vi "Manual Shooter Mode.vi"(8 "Shooter Angle":dbl format="%.2f", 10 "Manual Shoot":T1) -> (0 "Shooter Ready?":bool, 1 "Trigger Output":dbl, 2 "Right Output":dbl, 3 "Left Output":dbl, 4 "Angle Motor Out":dbl)   [LabVIEW 2015]
uses:
  Common Code/Manual Shoot.ctl
  Common Code/Change Detect Double.vi
  Robot Global Data.vi
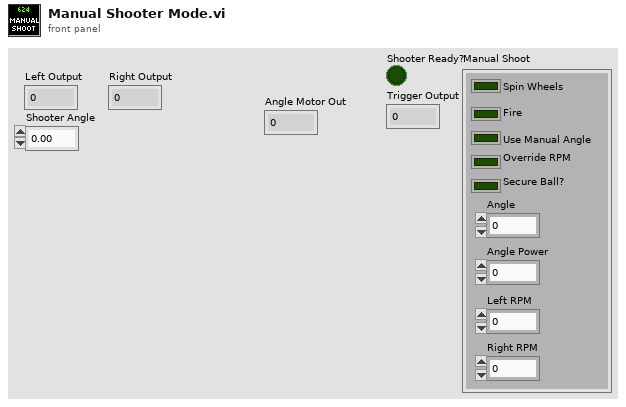
[diagram p1: front panel]
types:
  T1 = typedef "Manual Shoot.ctl" = cluster{"Spin Wheels":bool, "Fire":bool, "Angle":dbl, "Angle Power":dbl, "Use Manual Angle":bool, "Override RPM":bool, "Left RPM":dbl, "Right RPM":dbl, "Secure Ball?":bool}
  T2 = typedef "Dashboard Control Data.ctl" = cluster{"Shooter Presets":T3, "Encoder Control":T5, "Steer PID output":cluster{"output high":dbl, "output low":dbl}, " Steer PID gains":cluster{"proportional gain (Kc)":dbl, "integral time (Ti, min)":dbl, "derivative time (Td, min)":dbl}, "Drivetrain Settings":T6, "Vision Packet":T7, "Dashboard Drivetrain Command":T8, "Info/Command Cluster":T10, "Ball Vision Packet":T11, "Intake Presets":T13, "Intake Encoder Control":T15, "Climb Presets":T16, "Goal Output Range":cluster{"output high":dbl, "output low":dbl}, "Enabled Systems":T17, "Auton Presets":T18, "Pressure M":dbl, "Pressure B":dbl}
  T3 = typedef "Shooter Presets.ctl" = cluster{"Batter Shot":T4, "Deep Middle":T4, "Manual Shot":T4, "Left Ticks Per Rotation":dbl, "Right Ticks Per Rotation":dbl, "Low Bar Shot":T4, "Shooter RPM Tolerance":dbl, "Trigger Power":dbl, "Fire from Load Delay":i32, "Max Angle":dbl, "Min Angle":dbl, "Angle PID gains":cluster{"P":dbl, "I":dbl, "D":dbl}, "Angle Output":cluster{"output high":dbl, "output low":dbl}, "Shooter Angle Tolerance":dbl, "Vision Shoot x^2":dbl, "Vision Shoot x":dbl, "IR Let Go Timer":dbl, "Feed Forward Max Accel":dbl, "Feed Forward Kv":dbl, "Backwards Trigger":dbl, "Shot Finish Delay (ms)":dbl, "Angle Max Current":dbl, "Angle Current Trip Time":dbl, "Intake Angle":dbl, "Vision Shoot c":dbl, "Reset?":bool, "Button Release Delay":dbl, "Angle Pot x":dbl, "Angle Pot c":dbl, "Ignore Angle?":bool, "Max RPM":dbl, "Safty Frist Angle":dbl, "Intake Danger Height":dbl, "Angle Pot B":i32, "Angle Pot M":dbl, "FF Finish RPM":dbl, "RPM PID Right":cluster{"P":dbl, "I":dbl, "D":dbl, "FF":dbl}, "RPM PID Left":cluster{"P":dbl, "I":dbl, "D":dbl, "FF":dbl}, "Backwards RPM":dbl, "Vision RPM":dbl, "Run Wheels Backward Delay":u32, "Cleat Shot":T4}
  T4 = typedef "Shot Presets.ctl" = cluster{"L":dbl, "R":dbl, "A":dbl}
  T5 = typedef "Encoder Control.ctl" = cluster{"Right Tick Constant":dbl, "Left Tick Constant":dbl, "Reset?":bool, "Y Dist":cluster{"PID gains":cluster{"proportional gain (Kc)":dbl, "integral time (Ti, min)":dbl, "derivative time (Td, min)":dbl}}, "Y Stop Thresh":dbl, "Y Stop Speed":dbl}
  T6 = typedef "Drivetrain Settings.ctl" = cluster{"Gyro Tolerance":dbl, "Throttle Ramp (ms)":dbl, "Kv":dbl, "Ka":dbl, "Feed Forward P":dbl, "Feed Forward D":dbl, "Goal Vision PID gains":cluster{"proportional gain (Kc)":dbl, "integral time (Ti, min)":dbl, "derivative time (Td, min)":dbl}, "Goal Detection Window":dbl, "Creep Rate":dbl, "Vision Throttle Threshold":dbl, "Min Turn Output":dbl, "Left Batter Angle":dbl, "Right Batter Angle":dbl}
  T7 = typedef "Goal Vision Packet.ctl" = cluster{"Distance":dbl, "Center X":dbl, "Center Y":dbl, "Found Target?":bool, "Robot Center":dbl, "Angle":dbl}
  T8 = typedef "Dashboard Drivetrain Command.ctl" = cluster{"Drivetrain Vision":T9}
  T9 = typedef "Drivetrain Vision.ctl" = cluster{"Goal Window":dbl, "Ball Window":dbl}
  T10 = typedef "Ball Tracking Command Cluster.ctl" = cluster{"Distance to Ball":dbl, "Desired Angle":dbl, "Command":enum16{"Turn to Ball", "Turn to Angle", "Get Distance"}, "Pixels from Center":dbl}
  T11 = typedef "Ball Vision Packet.ctl" = cluster{"Ball Detected?":bool, "Distance to Ball":dbl, "Desired Angle":dbl, "Pixels from Center":dbl, "Tracking mode":T12}
  T12 = typedef "Tracking Mode.ctl" = enum16{"Turn to Ball", "Turn to Angle"}
  T13 = typedef "Intake Presets.ctl" = cluster{"Intake Speed":dbl, "Outake Speed":dbl, "Low Height":dbl, "Half Height":dbl, "Full Height":dbl, "Angle Speed":dbl, "Angle Tolerance":dbl, "Encoder Scale":dbl, "Load Height":dbl, "Output Range":T14, "Rotation Power Max/Min":dbl, "MaxCurrent":dbl, "Intake Trip Time":dbl, "Idle Height":dbl, "Max Height":dbl, "Reset Encoders?":bool, "PID gains":cluster{"proportional gain (Kc)":dbl, "integral time (Ti, min)":dbl, "derivative time (Td, min)":dbl}, "Intake Stop Delay":u32, "Settle Time":dbl, "Settle Wait Time":dbl}
  T14 = typedef "Drivetrain Output Range.ctl" = cluster{"output high":dbl, "output low":dbl}
  T15 = typedef "IntakeEcoderControl.ctl" = cluster{"Arm Tick Constant":dbl, "Reset?":bool, "Y Dist":cluster{"PID gains":cluster{"proportional gain (Kc)":dbl, "integral time (Ti, min)":dbl, "derivative time (Td, min)":dbl}}, "Y Stop Thresh":dbl, "Y Stop Speed":dbl}
  T16 = typedef "Climb Presets.ctl" = cluster{"Pull Power":dbl, "Extend Power":dbl}
  T17 = typedef "Enabled Systems.ctl" = cluster{"Shoot":bool, "Intake":bool, "DT":bool, "Gyro":bool, "100ms":bool, "US":bool}
  T18 = typedef "Autonomous Presets.ctl" = cluster{"Pitch Limit":dbl, "Roll Limit":dbl, "Start Position":dbl, "Cross Position":dbl}
  T19 = typedef "Intake Status Cluster.ctl" = cluster{"Roller Power":dbl, "Angle Power":dbl, "Intake Mode":T20, "Intake States":T21, "Rollers Active?":bool, "Current Height":dbl, "Target Height":dbl, "Encoder Raw Position":dbl, "Forward Tripped?":bool, "Backward Tripped?":bool, "Override IR?":bool}
  T20 = typedef "Intake Mode.ctl" = enum16{"Safe", "Auto", "Manual"}
  T21 = typedef "Intake States.ctl" = enum16{"Idle", "Set roller speed", "Move to angle", "Go Hard or Go Home", "Ball Settle"}
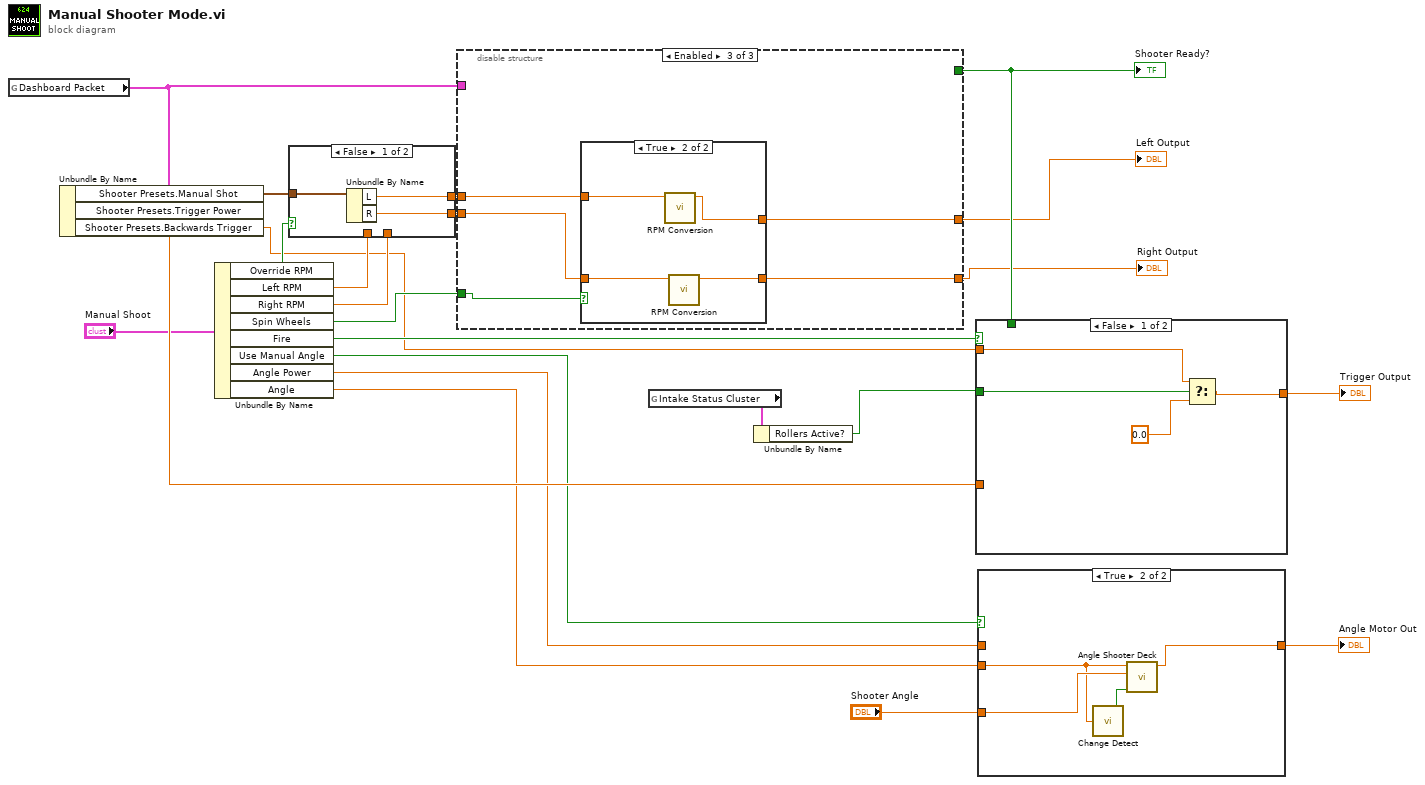
[diagram p0: block diagram]
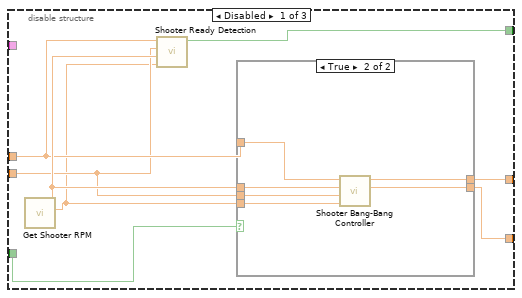
[diagram p2: hidden frame]
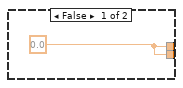
[diagram p3: hidden frame]
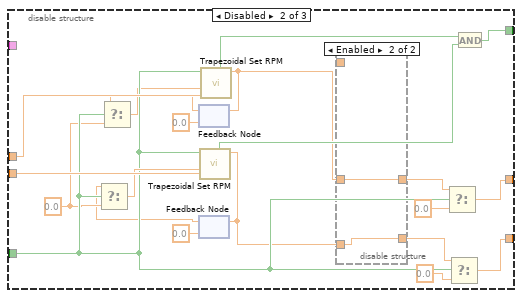
[diagram p4: hidden frame]
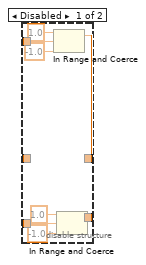
[diagram p5: hidden frame]
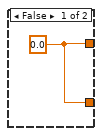
[diagram p6: hidden frame]
diagram:
  n1 = global read "Robot Global Data.vi" "Dashboard Packet"() -> (w2:T2)
  n2 = Unbundle By Name(w2) -> ("Shooter Presets.Manual Shot"=w23:T4, "Shooter Presets.Trigger Power"=w16:dbl, "Shooter Presets.Backwards Trigger"=w7:dbl)
  n3 = Unbundle By Name("Manual Shoot") -> ("Override RPM"=w11:bool, "Left RPM"=w10:dbl, "Right RPM"=w9:dbl, "Spin Wheels"=w22:bool, "Fire"=w8:bool, "Use Manual Angle"=w15:bool, "Angle Power"=w13:dbl, "Angle"=w12:dbl)
  n4 = case shown="False" w11 {
    tunnel: w23 -> [w26 _]
    tunnel: [w25 w28] -> w21
    tunnel: [w24 w27] -> w20
    tunnel: w10 -> [_ w28]
    tunnel: w9 -> [_ w27]
    frame False {
      n5 = Unbundle By Name(w26) -> ("L"=w25:dbl, "R"=w24:dbl)
    }
    frame True {
    }
  }
  n6 = disable-structure shown="Enabled" {
    disable-tunnel: w22 -> [w36 w50 w75]
    disable-tunnel: w21 -> [w34 w60 w79]
    disable-tunnel: w20 -> [w33 w61 w77]
    disable-tunnel: [w31 w64 _] -> w19
    disable-tunnel: [w30 w52 w78] -> w4
    disable-tunnel: [w29 w55 w76] -> w3
    disable-tunnel: w2 -> [_ _ _]
    frame Disabled {
      n7 = call "Get Shooter RPM.vi"() -> ("Right RPM"=w32:dbl, "Left RPM"=w35:dbl)  [unwired: 7 in, 3 out]
      n8 = call "Shooter Ready Detection.vi"("Right RPM"=w32, "Left RPM"=w35, "Right RPM Target"=w33, "Left RPM Target"=w34) -> ("Shooter Ready?"=w31:bool)  [unwired: 7 in]
      n9 = case shown="True" w36 {
        tunnel: w34 -> [_ w43]
        tunnel: w33 -> [_ w42]
        tunnel: [w37 w41] -> w30
        tunnel: [w37 w40] -> w29
        tunnel: w35 -> [_ w39]
        tunnel: w32 -> [_ w38]
        frame False {
          w37 = 0.0 ("Left Output Power")
        }
        frame True {
          n10 = call "Shooter Bang-Bang Controller.vi"("Right Current RPM"=w38, "Right Target RPM"=w42, "Left Current RPM"=w39, "Left Target RPM"=w43) -> ("Right Output Power"=w40:dbl, "Left Output Power"=w41:dbl)  [unwired: 6 in]
        }
      }
    }
    frame Disabled {
      w49 = 0.0 ("f")
      n11 = feedback #1(0.0 ("RPM")) -> (w46:dbl)
      n12 = Select(t=w46, s=w50, f=w49) -> (s? t:f=w47:dbl)
      n13 = feedback #2(0.0 ("RPM")) -> (w48:dbl)
      n14 = Select(t=w48, s=w50, f=w49) -> (s? t:f=w51:dbl)
      n15 = call "Trapezoidal Set RPM.vi"("Desired RPM"=w61, "Current RPM"=w51, "Spinning Wheels?"=w50) -> ("RPM"=w44:dbl, "Shooter Ready?"=w62:bool)  [unwired: 6 in, 1 out]
      n16 = feedback-in #2(w44) -> ()
      n17 = call "Trapezoidal Set RPM.vi"("Desired RPM"=w60, "Current RPM"=w47, "Spinning Wheels?"=w50) -> ("RPM"=w45:dbl, "Shooter Ready?"=w63:bool)  [unwired: 6 in, 1 out]
      n18 = feedback-in #1(w45) -> ()
      n19 = disable-structure shown="Enabled" {
        disable-tunnel: _ -> [w72 _]
        disable-tunnel: w44 -> [w67 w73]
        disable-tunnel: [w66 w73] -> w57
        disable-tunnel: [w65 w74] -> w54
        disable-tunnel: w45 -> [_ w74]
        frame Disabled {
          n20 = In Range and Coerce(upper limit=1.0, x=w72, lower limit=-1.0) -> (coerced(x)=w65:dbl)  [unwired: 1 out]
          n21 = In Range and Coerce(upper limit=1.0, x=w67, lower limit=-1.0) -> (coerced(x)=w66:dbl)  [unwired: 1 out]
        }
        frame Enabled {
        }
      }
      n22 = Select(t=w54, s=w50, f=0.0) -> (s? t:f=w52:dbl)
      n23 = Select(t=w57, s=w50, f=0.0) -> (s? t:f=w55:dbl)
      n24 = And(x=w63, y=w62) -> (x .and. y?=w64:bool)
    }
    frame Enabled {
      n25 = case shown="True" w75 {
        tunnel: w79 -> [_ w84]
        tunnel: [w80 w83] -> w78
        tunnel: w77 -> [_ w82]
        tunnel: [w80 w81] -> w76
        frame False {
          w80 = 0.0 ("RPM Out")
        }
        frame True {
          n26 = call "RPM Conversion.vi"("RPM"=w84) -> ("RPM Out"=w83:dbl)  [unwired: 10 in]
          n27 = call "RPM Conversion.vi"("RPM"=w82) -> ("RPM Out"=w81:dbl)  [unwired: 10 in]
        }
      }
    }
  }
  "Left Output" <- w4
  "Right Output" <- w3
  "Shooter Ready?" <- w19
  n28 = global read "Robot Global Data.vi" "Intake Status Cluster"() -> (w6:T19)
  n29 = Unbundle By Name(w6) -> ("Rollers Active?"=w17:bool)
  n30 = case shown="False" w8 {
    tunnel: w19 -> [_ _]
    tunnel: [w87 w89] -> w18
    tunnel: w17 -> [w85 _]
    tunnel: w16 -> [_ w89]
    tunnel: w7 -> [w86 _]
    frame False {
      n31 = Select(t=w86, s=w85, f=0.0 ("Trigger Output")) -> (s? t:f=w87:dbl)
    }
    frame True {
      # "Fire when Pressed"
    }
  }
  "Trigger Output" <- w18
  n32 = case shown="True" w15 {
    tunnel: [w90 w94] -> w14
    tunnel: w13 -> [w90 _]
    tunnel: w12 -> [_ w92]
    tunnel: "Shooter Angle" -> [_ w93]
    frame False {
    }
    frame True {
      n33 = call-poly "Change Detect.vi"("In"=w92) -> ("Changed?"=w91:bool)
      n34 = call "Angle Shooter Deck.vi"("reinitialize? (F)"=w91, "Shooter Angle"=w93, "Target Angle"=w92) -> ("Angle Motor Power Out"=w94:dbl)  [unwired: 8 in]
    }
  }
  "Angle Motor Out" <- w14
